vi "Init.vi"(0 "SPI Bus":T1=enum."Invalid", 11 "error in":errorcluster) -> (4 "comm interface out":refnum<class "Pixy Com.lvclass">, 15 "error out":errorcluster)   [LabVIEW 2018, in "RoboRIO SPI.lvclass"]
uses:
  RoboRIO SPI.lvclass
  <vilib>/Rock Robotics/SystemInterfaces/spilib/spi_bus.ctl
  library/Interface/Pixy Com.lvclass
  <vilib>/Rock Robotics/WPI/SPI/WPI_SPIMode.ctl
  C:/Users/David/Documents/GitHub/Pixy2LabVIEW/source/Interface/Pixy Com.lvclass
  RoboRIO SPI.lvclass/RoboRIO SPI.ctl
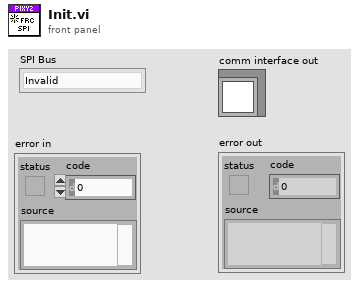
[diagram p1: front panel]
types:
  T1 = typedef "spi_bus.ctl" = enum16{"SPI On-Board, CS0", "SPI On-Board, CS1", "SPI On-Board, CS2", "SPI On-Board, CS3", "SPI MXP", "Invalid"}
  T2 = typedef "WPI_SPIMode.ctl" = enum16{"Mode 0 (Clk Idle Low,Sample on Leading)", "Mode 1 (Clk Idle Low,Sample on Trailing)", "Mode 2 (Clk Idle High,Sample on Leading)", "Mode 3 (Clk Idle High,Sample on Trailing)"}
  T3 = typedef "WPI_SPIDevRef.ctl" = cluster{"DevStatus":errorcluster, "Handle":i32, "SPI Bus":T1}
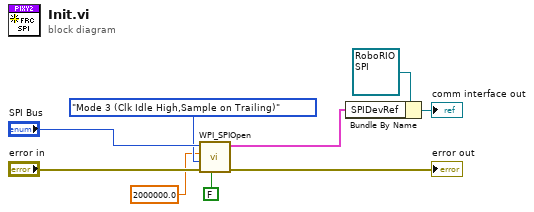
[diagram p0: block diagram]
diagram:
  n1 = call <vilib>:"WPI_SPIOpen.vi"("Chip Select Active High (F)"=FALSE, "error in"="error in", "Mode (3)"=WPI_SPIMode."Mode 3 (Clk Idle High,Sample on Trailing)", "Clock Rate (Hz)"=2000000.0, "SPI Bus"="SPI Bus") -> ("error out"=→"error out":errorcluster, "SPIDevRef"=w2:T3)  [unwired: 5 in]
  n2 = Bundle By Name(cluster=refnum<class "RoboRIO SPI.lvclass"> refnum ("comm interface out"), "SPIDevRef"=w2) -> (→"comm interface out":refnum<class "RoboRIO SPI.lvclass">)
